vi "PV Correction factor to string.vi"(1 "Input":sgl=1.0 min=0.2 max=9.9 step=0.1 format="%.2f") -> (0 "Output (String)":string)   [LabVIEW 2018, in "Pfeiffer Vacuum.lvlib"]
uses:
  <instrlib>/Pfeiffer Vacuum/Pfeiffer Vacuum.lvlib
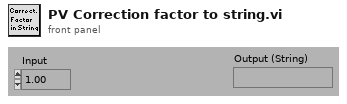
[diagram p1: front panel]
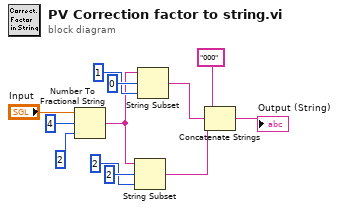
[diagram p0: block diagram]
diagram:
  n1 = Number To Fractional String(number="Input", width (-)=i16 4 ("Breite (-)"), precision (6)=i16 2 ("Genauigkeit (6)")) -> (F-format string=w4:string)  [unwired: 1 in]
  n2 = String Subset(string=w4, offset (0)=2 ("Offset (0)"), length (rest)=2 ("Länge")) -> (substring=w5:string)
  n3 = String Subset(string=w4, offset (0)=0 ("Offset (0)"), length (rest)=1 ("Länge")) -> (substring=w2:string)
  n4 = Concatenate Strings("000", w2, w5) -> (→"Output (String)":string)
